vi "IT-M3900C Output DC Volts.vi"() -> ()   [LabVIEW 2024]
doc: "This example shows how to configure the instrument's output voltage level, over current protection, and over voltage protection. The actual voltage level and actual current level are returned as well as whether over voltage protection (OVP) or over current protection (OCP) has been tripped."
uses:
  IT-M3900C.lvlib
panel:
  in  "Serial Configuration":T1={"Baud Rate"=9600, "Parity"=0, "Data Bits"=8, "Stop Bits"=10, "Flow Control"=0} {"Flow Control" items=["None", "XON/XOFF", "RTS/CTS", "XON/XOFF & RTS/CTS", "DTR/DSR", "XON/XOFF & DTR/DSR"]; "Stop Bits" items=["1.0"=10, "1.5"=15, "2.0"=20]; "Data Bits" items=["7"=7, "8"=8]; "Parity" items=["None", "Odd", "Even", "Mark", "Space"]; "Baud Rate" items=["300"=300, "600"=600, "1200"=1200, "2400"=2400, "4800"=4800, "9600"=9600, "19200"=19200, "38400"=38400, "57600"=57600, "115200"=115200]}
  in  "OCP Delay(S)":dbl min=0.0 max=60.0
  in  "OVP Delay(S)":dbl min=0.0 max=60.0
  in  "Current Limit (A)":dbl
  in  "Enable OCP":bool
  in  "Enable OVP":bool
  in  "Stop Output":bool
  in  "OVP Level (V)":dbl format="%.2f"
  out "Actual Current Limit (A)":dbl format="%.2f"
  out "Actual Voltage Level (V)":dbl format="%.2f"
  in  "Voltage Level (V)":dbl format="%.2f"
  in  "OCP Level (A)":dbl format="%.2f"
  in  "VISA resource name":refnum<visa-resource-name>
  # "(c) 2014 <Enter Company Name Here>.  ALL RIGHTS RESERVED."
  # "Over Voltage Protection"
  # "Over Current Protection"
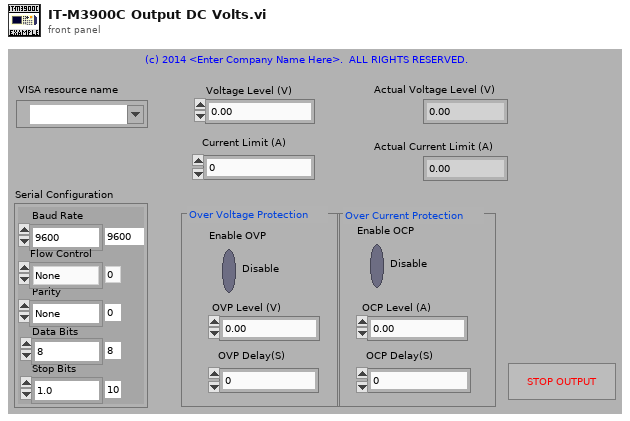
[diagram p1: front panel]
types:
  T1 = cluster{"Baud Rate":u32, "Parity":u16, "Data Bits":u16, "Stop Bits":u16, "Flow Control":u16}
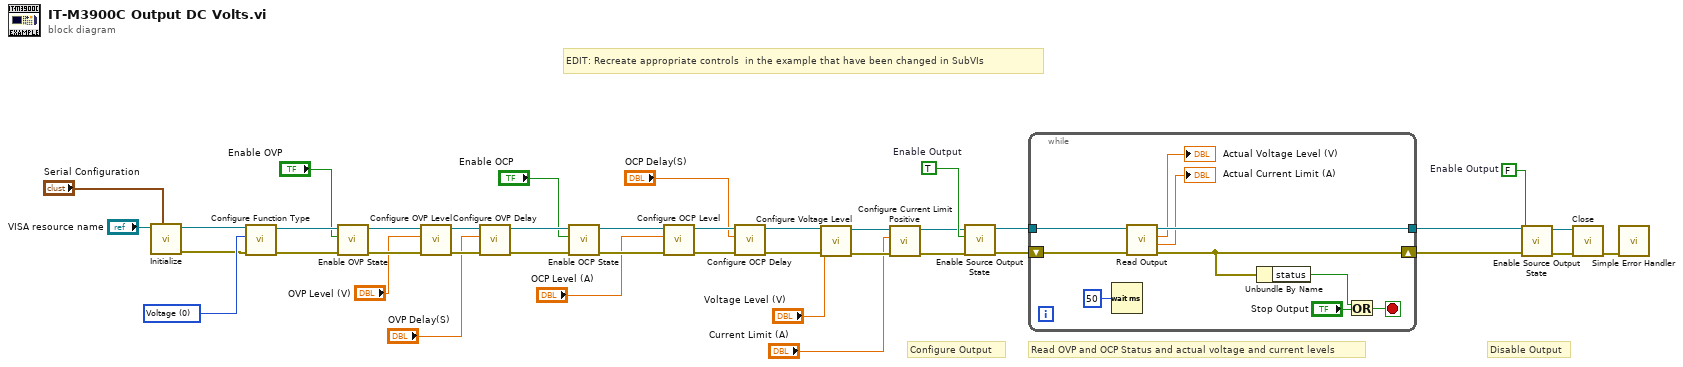
[diagram p0: block diagram]
diagram:
  w30 = u16 0 items=["Voltage", "Current"] ("Type")
  w33 = FALSE  # Enable Output
  w31 = TRUE  # Enable Output
  # "EDIT: Recreate appropriate controls  in the example that have been changed in SubVIs"
  # "Disable Output"
  # "Read OVP and OCP Status and actual voltage and current levels"
  # "Configure Output"
  n1 = call "Initialize.vi"("Serial Configuration"="Serial Configuration", "VISA resource name"="VISA resource name") -> ("error out"=w29:errorcluster, "VISA resource name out"=w28:refnum<visa-resource-name>)  [unwired: 8 in]
  n2 = call "Configure Function Type.vi"("error in"=w29, "Type"=w30, "VISA resource name"=w28) -> ("error out"=w26:errorcluster, "VISA resource name out"=w27:refnum<visa-resource-name>)  [unwired: 7 in]
  n3 = call "Enable OVP State.vi"("error in"=w26, "State"="Enable OVP", "VISA resource name"=w27) -> ("error out"=w24:errorcluster, "VISA resource name out"=w25:refnum<visa-resource-name>)  [unwired: 7 in]
  n4 = call "Configure OVP Level.vi"("error in"=w24, "Level(V)"="OVP Level (V)", "VISA resource name"=w25) -> ("error out"=w22:errorcluster, "VISA resource name out"=w23:refnum<visa-resource-name>)  [unwired: 7 in]
  n5 = call "Configure OVP Delay.vi"("error in"=w22, "Delay(S)"="OVP Delay(S)", "VISA resource name"=w23) -> ("error out"=w20:errorcluster, "VISA resource name out"=w21:refnum<visa-resource-name>)  [unwired: 7 in]
  n6 = call "Enable OCP State.vi"("error in"=w20, "State"="Enable OCP", "VISA resource name"=w21) -> ("error out"=w18:errorcluster, "VISA resource name out"=w19:refnum<visa-resource-name>)  [unwired: 7 in]
  n7 = call "Configure OCP Level.vi"("error in"=w18, "Level(A)"="OCP Level (A)", "VISA resource name"=w19) -> ("error out"=w16:errorcluster, "VISA resource name out"=w17:refnum<visa-resource-name>)  [unwired: 7 in]
  n8 = call "Configure OCP Delay.vi"("error in"=w16, "Delay(S)"="OCP Delay(S)", "VISA resource name"=w17) -> ("error out"=w8:errorcluster, "VISA resource name out"=w9:refnum<visa-resource-name>)  [unwired: 7 in]
  n9 = call "Configure Voltage Level.vi"("error in"=w8, "Voltage(V)"="Voltage Level (V)", "VISA resource name"=w9) -> ("error out"=w6:errorcluster, "VISA resource name out"=w7:refnum<visa-resource-name>)  [unwired: 7 in]
  n10 = call "Configure Current Limit Positive.vi"("error in"=w6, "Value(A)"="Current Limit (A)", "VISA resource name"=w7) -> ("error out"=w4:errorcluster, "VISA resource name out"=w5:refnum<visa-resource-name>)  [unwired: 7 in]
  n11 = call "Enable Source Output State.vi"("error in"=w4, "State"=w31, "VISA resource name"=w5) -> ("error out"=w38:errorcluster, "VISA resource name out"=w39:refnum<visa-resource-name>)  [unwired: 7 in]
  n12 = while {
    tunnel: w39 -> [w49]
    tunnel: [w50] -> w37
    shift-right: [w43] -> w36
    shift-left: w38 -> [w48]
    stop <- w45 stop-if-true
    n13 = Wait (ms)(milliseconds to wait=u32 50 ("等待时间（毫秒）")) -> ()  [unwired: 1 out]
    n14 = call "Read Output.vi"("error in"=w48, "VISA resource name"=w49) -> ("error out"=w43:errorcluster, "Actual Current Level (A)"=→"Actual Current Limit (A)":dbl, "Actual Voltage Level (V)"=→"Actual Voltage Level (V)":dbl, "VISA resource name out"=w50:refnum<visa-resource-name>)  [unwired: 6 in]
    n15 = Unbundle By Name(w43) -> ("status"=w42:bool)
    n16 = Or(x=w42, y="Stop Output") -> (x .or. y?=w45:bool)
  }
  n17 = call "Enable Source Output State.vi"("error in"=w36, "State"=w33, "VISA resource name"=w37) -> ("error out"=w34:errorcluster, "VISA resource name out"=w35:refnum<visa-resource-name>)  [unwired: 7 in]
  n18 = call "Close.vi"("error in"=w34, "VISA resource name"=w35) -> ("error out"=w32:errorcluster)  [unwired: 9 in]
  n19 = call <vilib>:"Simple Error Handler.vi"("error in (no error)"=w32) -> ()  [unwired: 4 in, 5 out]
